vi "Program_Active_server.vi"(0 "Client Name":string, 1 "Client Messages":string, 2 "Traverse level State":T1, 3 "Mode":enum16{"Program Active", "Traverse Level State"}(ring), 4 "People to Email":string[](array[string]), 8 "Time till next contact (Sec)":dbl format="%.2f") -> ()   [LabVIEW 2017]
uses:
  ADAM Client/Sub VIs/ADAM Controls/Traverse_Level_State.ctl
  ADAM Client/Sub VIs/ADAM Controls/Module_type_ADAM.ctl
  ADAM Client/Sub VIs/ADAM Controls/Channel_State.ctl
  ADAM Client/Sub VIs/ADAM Controls/Ch_description_ADAM.ctl
  ADAM Client/Sub VIs/ADAM Controls/Function_ADAM.ctl
  ADAM Client/Sub VIs/ADAM Controls/Calib_type_ADAM.ctl
  ADAM Client/Sub VIs/ADAM Controls/Address.ctl
  ADAM_Global.vi
  Anemometry/Anemometry Sub Vis/Globals/Preference_global.vi
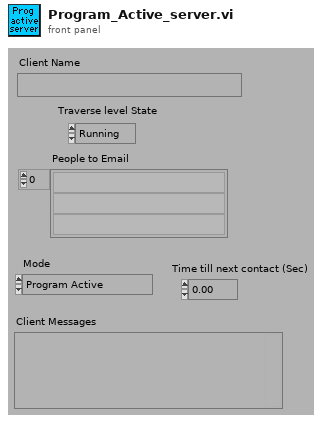
[diagram p1: front panel]
types:
  T1 = typedef "Traverse_Level_State.ctl" = enum16{"Running", "Complete"}
  T2 = typedef "Calib_type_ADAM.ctl" = string
  T3 = typedef "Ch_description_ADAM.ctl" = cluster{"Ch Name":string, "Type":T4, "Function":T5, "Ch State":T6, "Calibration type":T2, "A":dbl, "B":dbl, "C":dbl, "D":dbl, "Comments":string, "Address":T7, "String":string, "Duty":u16}
  T4 = typedef "Module_type_ADAM.ctl" = string
  T5 = typedef "Function_ADAM.ctl" = enum16{"Analogue Input", "Digital Input", "Event counter", "Event rate", "Analogue Output", "Digital Output", "Relay Output"}
  T6 = typedef "Channel_State.ctl" = enum16{"On", "Off", "Always On", "Always Off"}
  T7 = typedef "Address.ctl" = cluster{"Main":i32, "Ch.":i32, "Sub":i32, "Port Name":string}
  T8 = enum16{"Append to Global", "Read Global then Clear"}
  T9 = typedef "Client_State_Cluster.ctl" = cluster{"Client Name":string, "Traverse level State":T1, "People to Email":string[], "Next Contact Time":dbl}
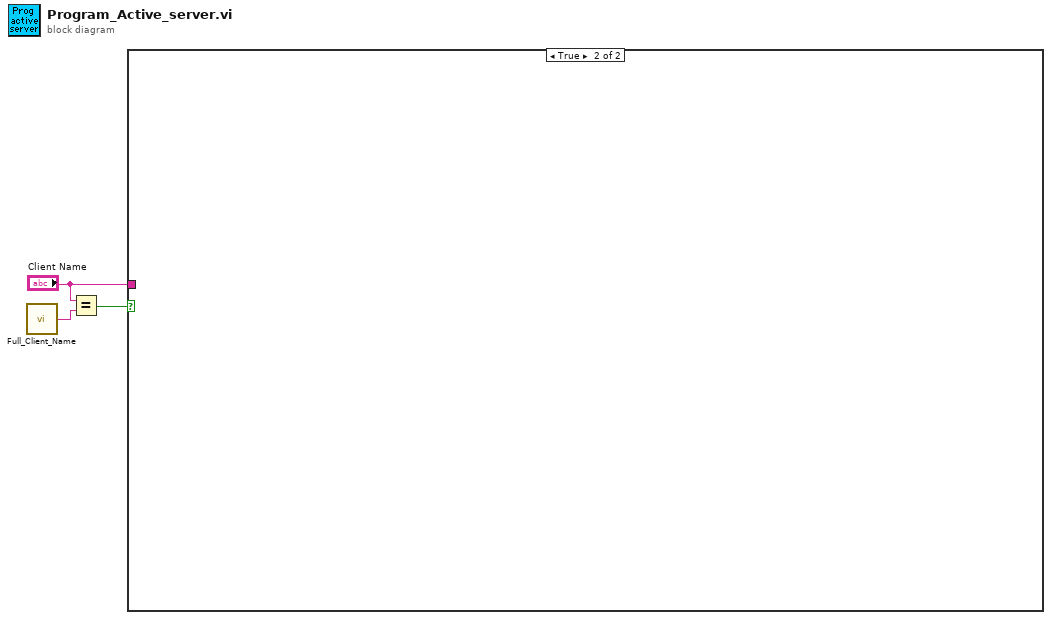
[diagram p0: block diagram]
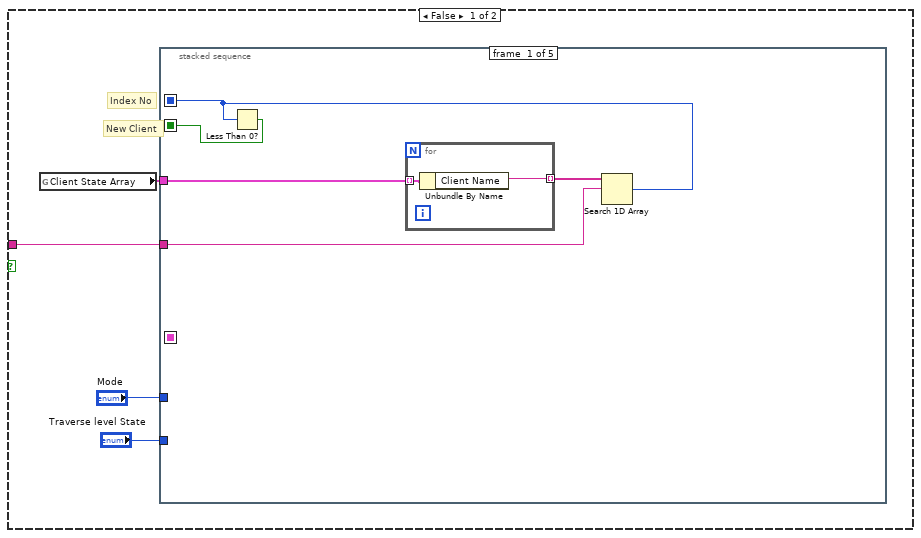
[diagram p2: hidden frame]
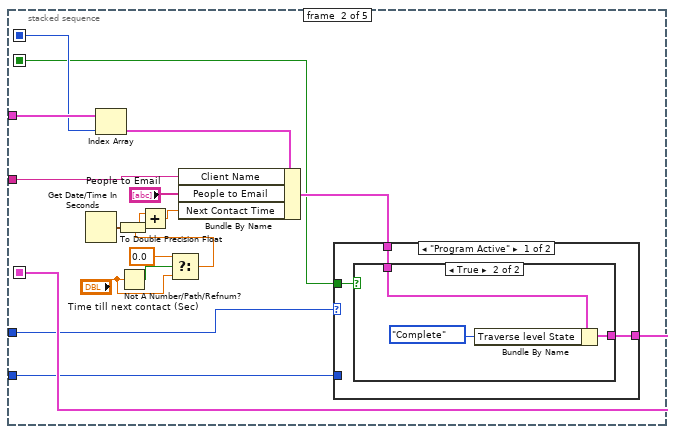
[diagram p3: hidden frame]
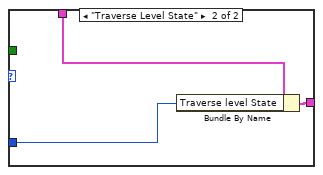
[diagram p5: hidden frame]
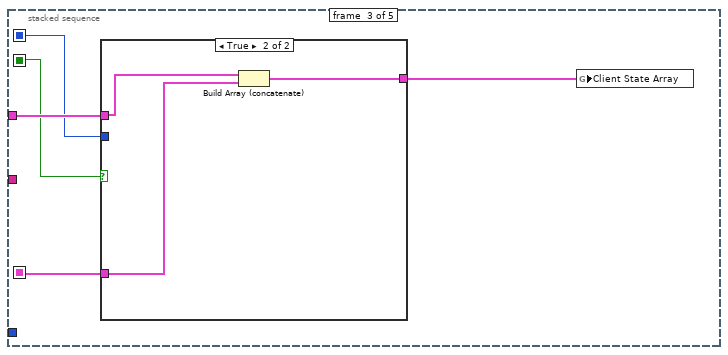
[diagram p6: hidden frame]
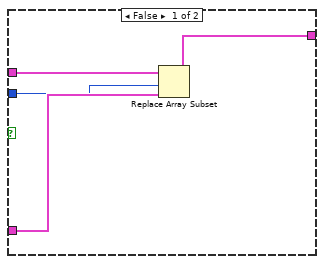
[diagram p7: hidden frame]
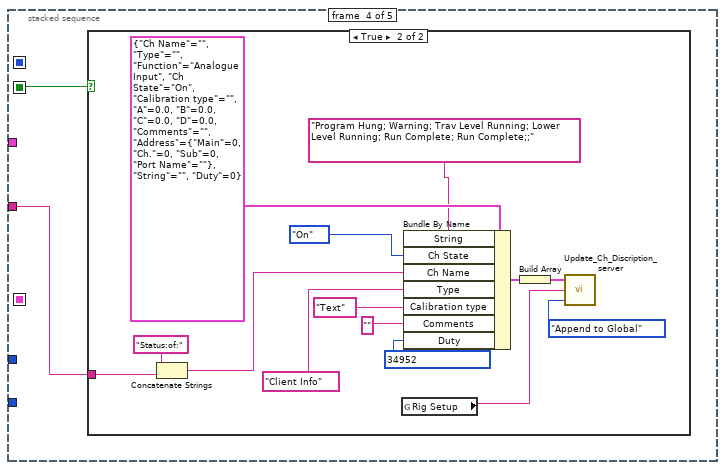
[diagram p8: hidden frame]
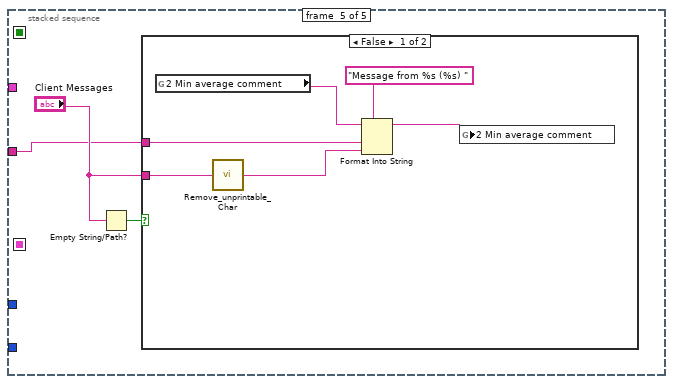
[diagram p10: hidden frame]
diagram:
  n1 = call "Full_Client_Name.vi"() -> ("Client Name"=w2:string)
  n2 = Equal?(x="Client Name", y=w2) -> (x = y?=w1:bool)
  n3 = case shown="True" w1 {
    tunnel: "Client Name" -> [w4 _]
    frame False {
      # "New Client"
      # "Index No"
      n4 = global read "ADAM_Global.vi" "Client State Array"() -> (w7:T9[])
      n5 = stacked-sequence {
        seq-local: [_ w28 _ _ _] -> [_ _ w45 _ _]
        seq-local: [w10 _ _ _ _] -> [_ w26 w43 _ _]
        seq-local: [w9 _ _ _ _] -> [_ w25 w42 w54 _]
        tunnel: w7 -> [w11 w31 w46 _ _]
        tunnel: "Mode" -> [_ w24 _ _ _]
        tunnel: "Traverse level State" -> [_ w23 _ _ _]
        tunnel: w4 -> [w8 w22 _ w55 w70]
        frame #0 {
          n6 = for {
            tunnel: w11 -> [w14] mode=indexing
            tunnel: [w13] -> w12 mode=indexing
            n7 = Unbundle By Name(w14) -> ("Client Name"=w13:string)
          }
          n8 = Search 1D Array(1D array=w12, element=w8) -> (index of element=w10:i32)  [unwired: 1 out]
          n9 = Less Than 0?(x=w10) -> (x < 0?=w9:bool)
        }
        frame #1 {
          n10 = Get Date/Time In Seconds() -> (seconds since 1Jan1904=w15:timestamp)
          n11 = Index Array(array=w31, index=w26) -> (element=w30:T9)
          n12 = To Double Precision Float(number=w15) -> (double precision float=w21:dbl)
          n13 = Not A Number/Path/Refnum?(number/path/refnum="Time till next contact (Sec)") -> (NaN/Path/Refnum?=w19:bool)
          n14 = Select(t=0.0, s=w19, f="Time till next contact (Sec)") -> (s? t:f=w16:dbl)
          n15 = Add(x=w21, y=w16) -> (x+y=w20:dbl)
          n16 = Bundle By Name(cluster=w30, "Client Name"=w22, "People to Email"="People to Email", "Next Contact Time"=w20) -> (w29:T9)
          n17 = case shown="\"Program Active\"" w24 {
            tunnel: w29 -> [w33 w41]
            tunnel: [w32 w40] -> w28
            tunnel: w25 -> [w34 _]
            tunnel: w23 -> [_ w39]
            frame "Program Active" {
              n18 = case shown="True" w34 {
                tunnel: w33 -> [w35 w38]
                tunnel: [w35 w37] -> w32
                frame False {
                }
                frame True {
                  n19 = Bundle By Name(cluster=w38, "Traverse level State"=Traverse_Level_State."Complete" ("Bundle Element")) -> (w37:T9)
                }
              }
            }
            frame "Traverse Level State" {
              n20 = Bundle By Name(cluster=w41, "Traverse level State"=w39) -> (w40:T9)
            }
          }
        }
        frame #2 {
          n21 = case shown="True" w42 {
            tunnel: w46 -> [w50 w51]
            tunnel: w45 -> [w48 w53]
            tunnel: [w49 w52] -> w44
            tunnel: w43 -> [w47 _]
            frame False {
              n22 = Replace Array Subset(array=w50, new element=w48, index=w47) -> (w49:T9[])
            }
            frame True {
              n23 = Build Array (concatenate)(w51, w53) -> (w52:T9[])
            }
          }
          n24 = global write "ADAM_Global.vi" "Client State Array"(w44) -> ()
        }
        frame #3 {
          n25 = case shown="True" w54 {
            tunnel: w55 -> [_ w60]
            frame False {
            }
            frame True {
              n26 = Concatenate Strings("Status:of:", w60) -> (w59:string)
              n27 = global read "Preference_global.vi" "Rig Setup"() -> (w58:string)
              n28 = Bundle By Name(cluster=T3 {"Ch Name"="", "Type"="", "Function"=enum."Analogue Input", "Ch State"=enum."On", "Calibration type"="", "A"=0.0, "B"=0.0, "C"=0.0, "D"=0.0, "Comments"="", "Address"={"Main"=0, "Ch."=0, "Sub"=0, "Port Name"=""}, "String"="", "Duty"=0} ("Ch Discription"), "String"="Program Hung; Warning; Trav Level Running; Lower Level Running; Run Complete; Run Complete;;", "Ch State"=Channel_State."On", "Ch Name"=w59, "Type"=T4 "Client Info", "Calibration type"=T2 "Text", "Comments"="" ("Substring"), "Duty"=u16 34952 ("Bundle Element")) -> (w68:T3)
              n29 = Build Array(w68) -> (w67:T3[])
              n30 = call "Update_Ch_Discription_server.vi"("Mode"=T8."Append to Global", "Client HD name"=w58, "Channels to update In"=w67) -> ()  [unwired: 1 out]
            }
          }
        }
        frame #4 {
          n31 = Empty String/Path?(string/path="Client Messages") -> (empty?=w72:bool)
          n32 = case shown="False" w72 {
            tunnel: "Client Messages" -> [w78 _]
            tunnel: w70 -> [w76 _]
            frame False {
              n33 = global read "ADAM_Global.vi" "2 Min average comment"() -> (w77:string)
              n34 = call "Remove_unprintable_Char.vi"("Input String"=w78) -> ("Output String"=w75:string)
              n35 = Format Into String(format string="Message from %s (%s) ", initial string=w77, w76, w75) -> (resulting string=w73:string)  [unwired: 1 in, 1 out]
              n36 = global write "ADAM_Global.vi" "2 Min average comment"(w73) -> ()
            }
            frame True {
            }
          }
        }
      }
    }
    frame True {
    }
  }
